vi "ecg_ncs_v3.vi"() -> ()   [LabVIEW 2016]
uses:
  <instrlib>/niUSRP/niUSRP Timestamp.ctl
  C:/Program Files/National Instruments/LabVIEW 2016/examples/Instrument IO/Serial/support/Serial - Settings.ctl
  State.ctl
  <vilib>/Instr/_visa.llb/VISA Configure Serial Port (Instr).vi
  <instrlib>/niUSRP/niUSRP Write Tx Data (2D CDB).vi
  <instrlib>/niUSRP/niUSRP Fetch Rx Data (2D CDB).vi
panel:
  in  "File Name 2":string="Test"
  in  "Path 2":path=path "D:/Research/SummerFall17Spring18/CnC/NCS/EcgNcsCorrelation/Labview Codes/ECG_NCS"
  out "#Loop = #Packets Received":i32
  out "ECGsample":i16
  out "PhNcs":dbl
  out "AmpNcs":dbl
  out "AmpNcsDS":dbl
  out "PhNcsDS":dbl
  out "error IO 2":errorcluster={"status"=FALSE, "code"=-1074118647, "source"=""}
  in  "Serial Settings":T1={"baud rate"=57600, "data bits"=8, "parity"=enum."None", "stop bits"=10, "flow control"=0} {"flow control" items=["None"=0, "XON/XOFF"=1, "RTS/CTS"=2, "DTR/DSR"=4]; "stop bits" items=["1.0"=10, "1.5"=15, "2.0"=20]; "data bits" min=5 max=8 step=1; "baud rate" items=["75"=75, "110"=110, "134"=134, "150"=150, "300"=300, "600"=600, "1200"=1200, "1800"=1800, "2400"=2400, "4800"=4800, "7200"=7200, "9600"=9600, "14400"=14400, "19200"=19200, "28800"=28800, "38400"=38400, "56000"=56000, "57600"=57600, "115200"=115200, "128000"=128000, "230400"=230400]}
  in  "VISA resource name":refnum<visa-resource-name>="bmd101"
  out "ECG":i16(graph)
  in  "byte count":u32=1
  out "Coerced Rx IQ Rate":dbl
  in  "Sampling Rate":i32=500
  out "Gain":dbl=-15.0
  out "Bandwidth":dbl=56000000.0
  out "Coerced Carrier Frequency":dbl=2000000000.0 format="%#.17g"
  out "Coerced Tx IQ rate":dbl=1000000.0
  out "error IO":errorcluster={"status"=FALSE, "code"=-1074118647, "source"=""}
  in  "Rx Number of Samples":i32=10000
  in  "Tab Control 2":enum32{"NI-294x/295x", "NI-2900/2901"}(tab)=enum."NI-2900/2901"
  in  "Rx carrier frequency [Hz]":dbl=2000000000.0 format="%#_6p"
  in  "Tx carrier frequency [Hz]":dbl=1000000000.0 format="%#_6p"
  in  "Start Trigger Time":T2={"whole seconds"=1, "fractional seconds"=0.0}
  in  "Tab Control":T3(tab)
  out "NCS tag Amp":dbl[](graph)=[0.011967714738528729, 0.012021355192189592, 0.012015275039596582, 0.011969166030167903, 0.011958890166168242, 0.012007893820858737, 0.012022893722444085, 0.011978222225113794, 0.011969989939463181, 0.012003099640895068]
  out "NCS tag Phase":dbl[](graph)=[0.011967714738528729, 0.012021355192189592, 0.012015275039596582, 0.011969166030167903, 0.011958890166168242, 0.012007893820858737, 0.012022893722444085, 0.011978222225113794, 0.011969989939463181, 0.012003099640895068]
  out "Tag Amp":dbl[](graph)
  out "Tag Phase":dbl[](graph)
  out "Tx Waveform Graph":waveform(dbl)[](graph)
  in  "Stop":bool
  in  "Channel 0\nTone Amplitude":dbl=0.707 step=0.05 format="%#.6g"
  in  "Channel 0 \nTone Frequency":dbl=5000.0 format="%#_6p"
  in  "Tx Waveform Size":dbl=2000.0
  in  "Device Name":refnum<k15>="MyB200"
  in  "Tx Gain":dbl=28.0 format="%#_6f"
  in  "Tx IQ Rate":dbl=1000000.0 format="%#_6p"
  in  "Rx Gain":dbl=32.0 format="%#_6f"
  in  "Rx IQ Rate":dbl=1000000.0 format="%#_6p"
  # "Rx Settings"
  # "Tx Settings"
  # "Note that on the NI-2900 and NI-2901, both Rx channels share an LO and both Tx channels share an LO. However, on the NI-294x/295x devices, Rx and Tx of channel 0 share an LO and Rx and Tx of channel 1 share an LO."
  # "Rx: Number of samples should be 1e6/512 in one loop."
  # "This Tx graph should always have end and start tied up since this is being sent in a loop continuously. Otherwise phase jumps will be noticed."
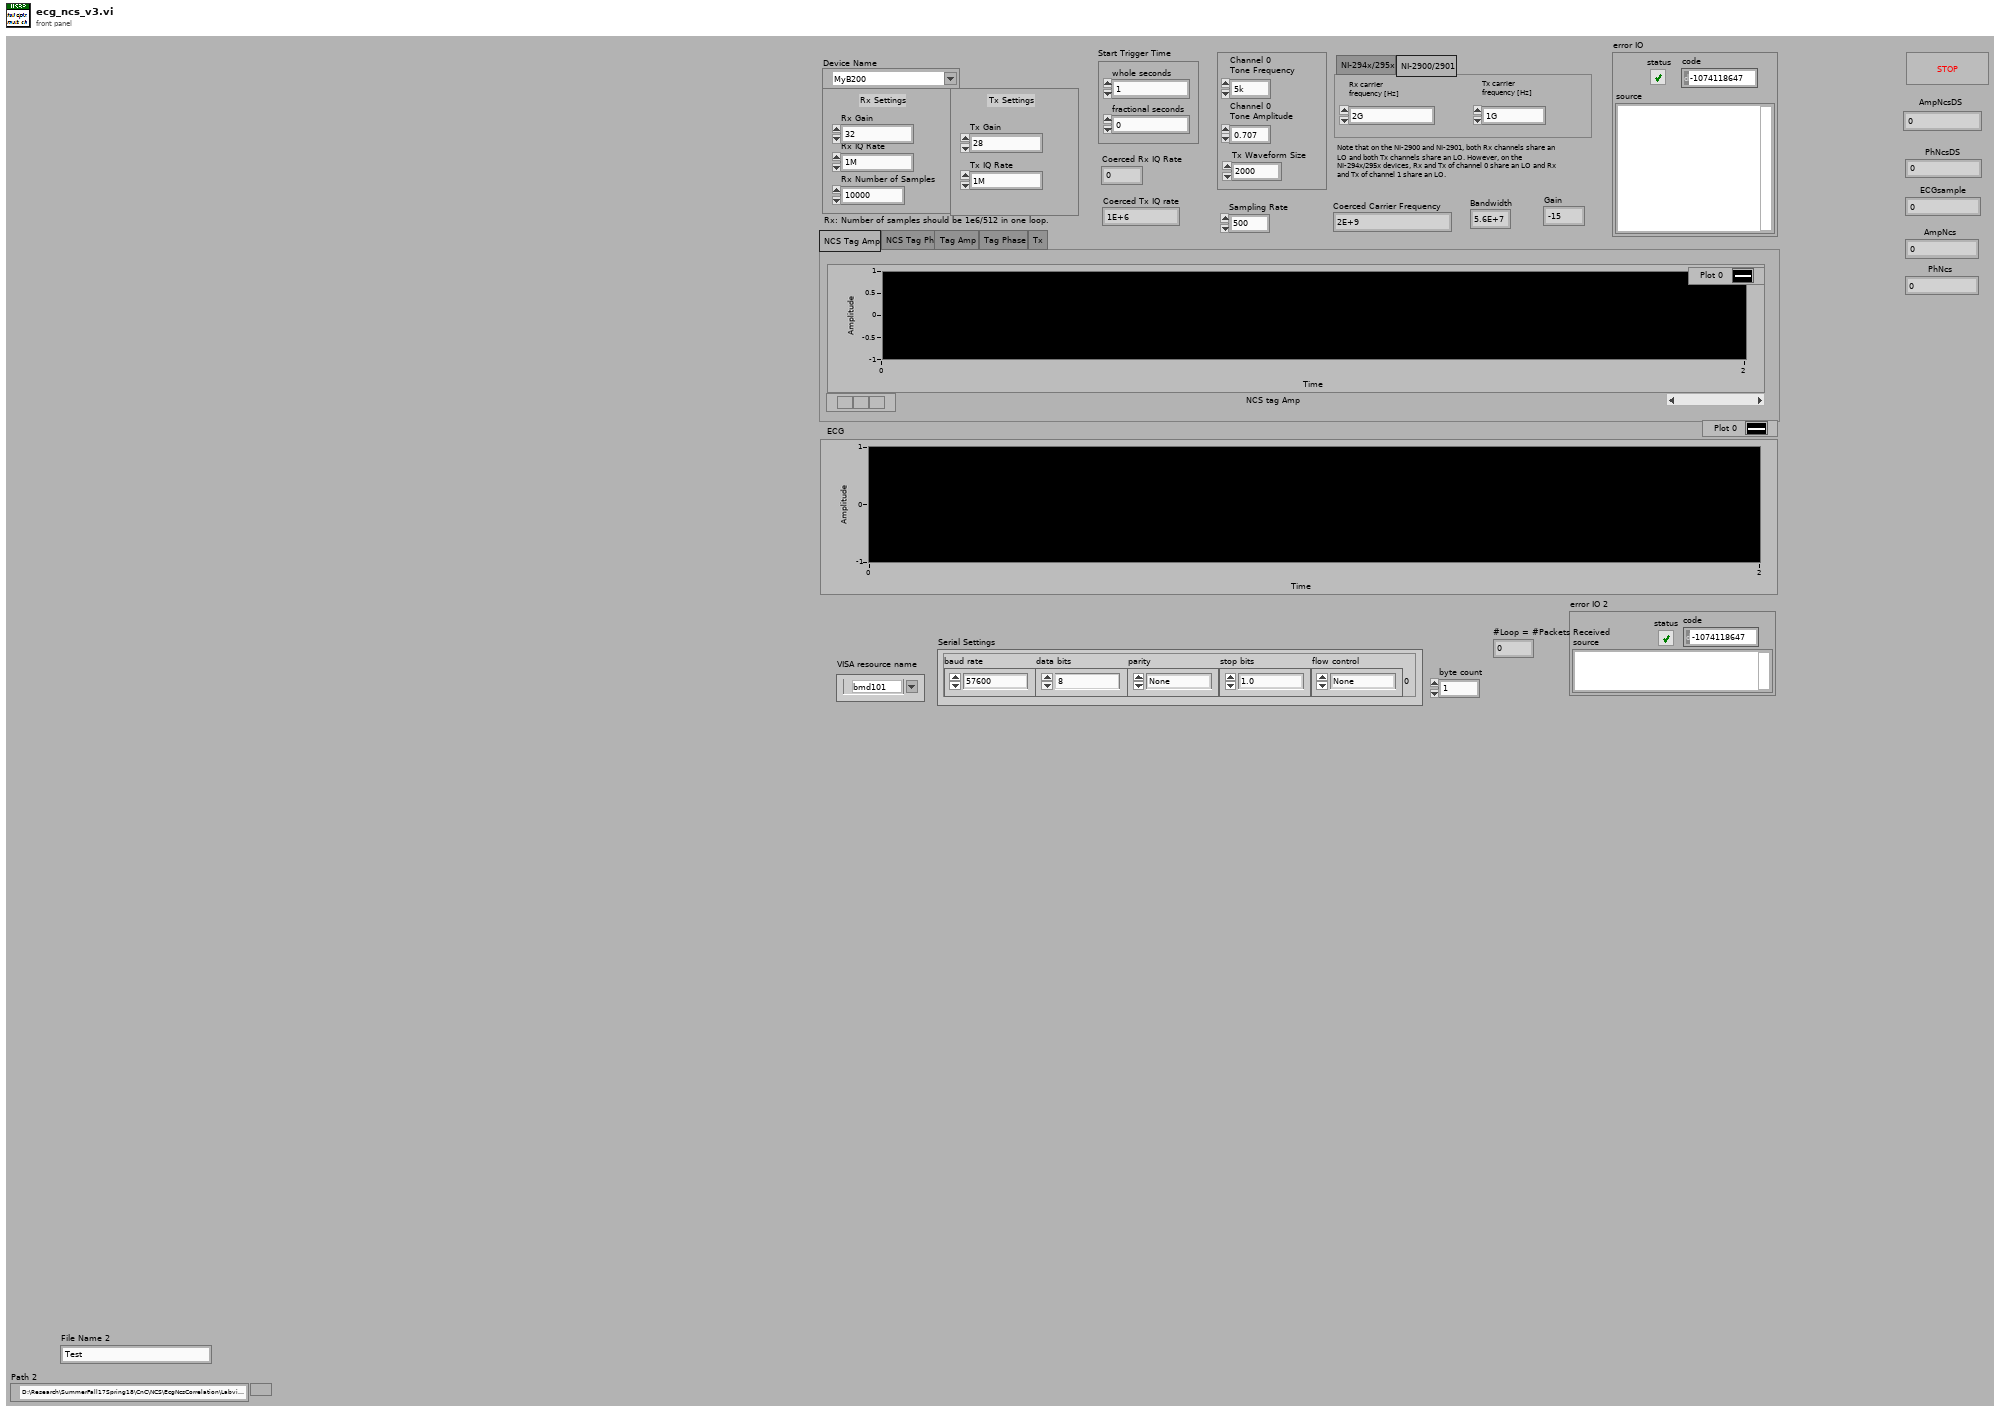
[diagram p1: front panel]
types:
  T1 = typedef "Serial - Settings.ctl" = cluster{"baud rate":u32, "data bits":u16, "parity":enum16{"None", "Odd", "Even", "Mark", "Space"}, "stop bits":u16, "flow control":u16}
  T2 = typedef "niUSRP Timestamp.ctl" = cluster{"whole seconds":u64, "fractional seconds":dbl}
  T3 = enum32{"NCS Tag Amp", "NCS Tag Ph", "Tag Amp", "Tag Phase", "Tx"}
  T4 = typedef "State.ctl" = enum16{"Initialize", "get byte", "check", "packet received", "packet approved"}
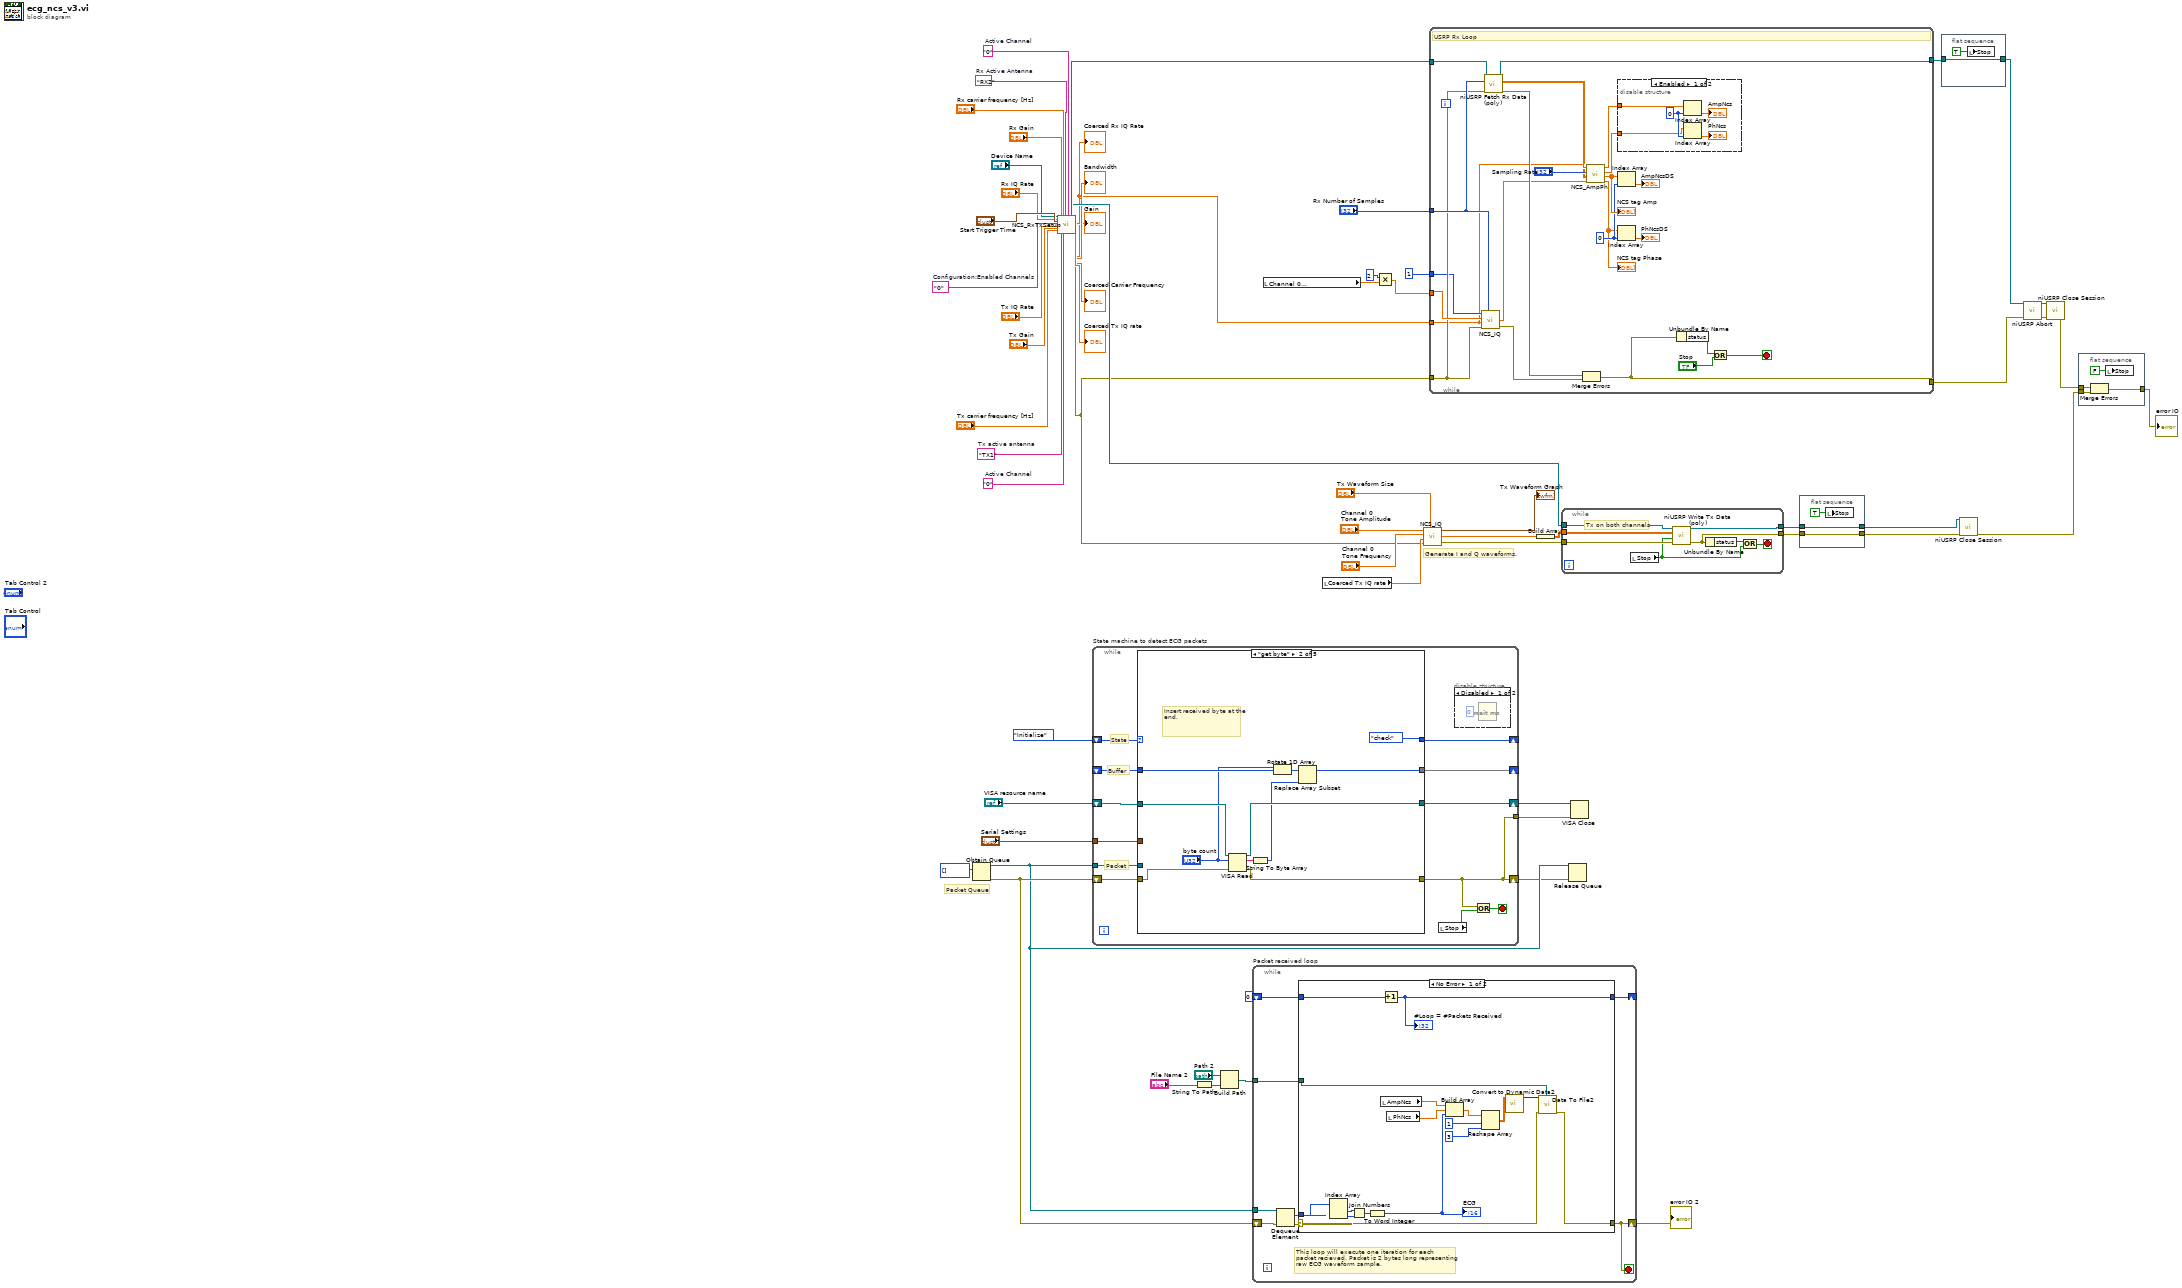
[diagram p0: block diagram]
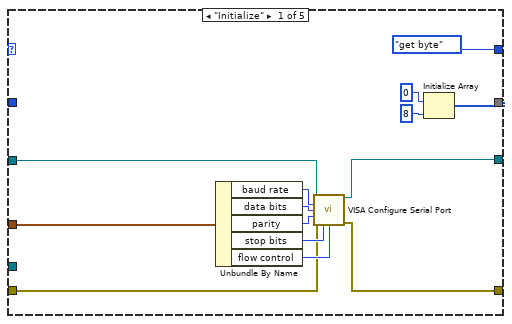
[diagram p4: hidden frame]
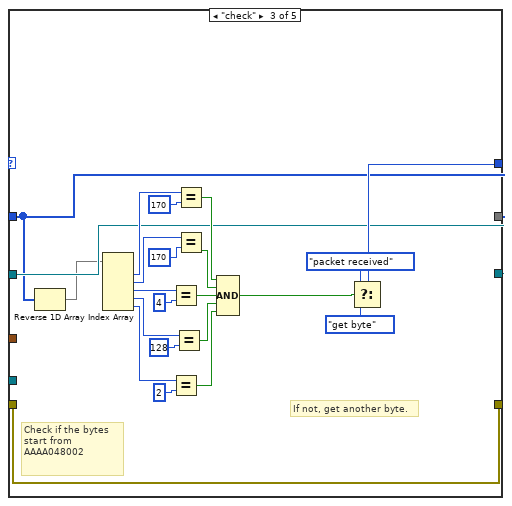
[diagram p5: hidden frame]
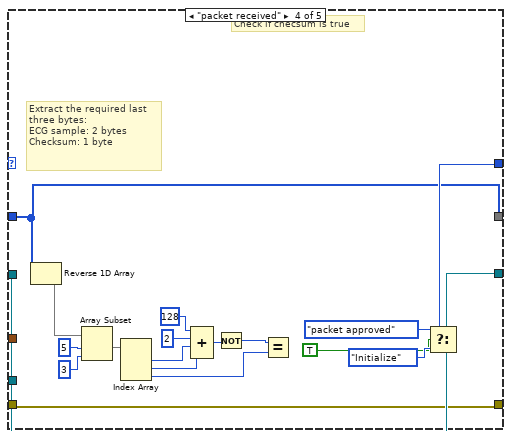
[diagram p6: hidden frame]
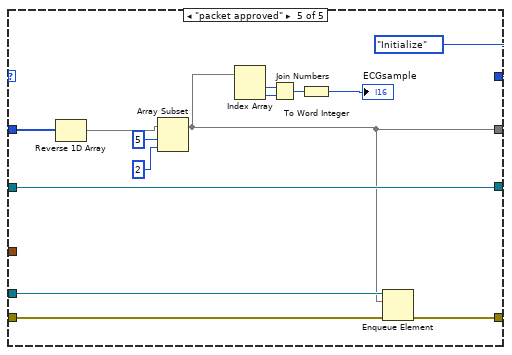
[diagram p7: hidden frame]
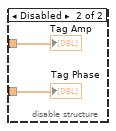
[diagram p8: hidden frame]
diagram:
  w17 = "0"  # Active Channel
  w18 = "0"  # Active Channel
  w53 = "RX2"  # Rx Active Antenna
  w49 = "TX1"  # Tx active antenna
  w35 = "0"  # Configuration:Enabled Channels
  # "Packet Queue"
  # "Generate I and Q waveforms."
  n1 = Obtain Queue(element data type=u8[] []) -> (queue out=w12:refnum<queue>, error out=w13:errorcluster)  [unwired: 4 in, 1 out]
  n2 = call "NCS_RxTxSetup.vi"("IVI Refnum in"="Device Name", "Rx IQ Rate"="Rx IQ Rate", "Start Trigger Time"="Start Trigger Time", "Configuration:Enabled Channels"=w35, "Tx IQ Rate"="Tx IQ Rate", "Tx Gain"="Tx Gain", "Tx carrier frequency [Hz]"="Tx carrier frequency [Hz]", "Rx Gain"="Rx Gain", "Tx active antenna"=w49, "Rx carrier frequency [Hz]"="Rx carrier frequency [Hz]", "Active Channel"=w17, "Rx Active Antenna"=w53, "Active Channel 2"=w18) -> ("session handle out"=w60:refnum<k15>, "IVI Refnum out"=w61:refnum<k15>, "Coerced Rx IQ Rate"=w16:dbl, "Bandwidth"=→"Bandwidth":dbl, "Gain"=→"Gain":dbl, "Carrier Frequency"=→"Coerced Carrier Frequency":dbl, "IQ Rate 2"=→"Coerced Tx IQ rate":dbl, "error out"=w28:errorcluster)  [unwired: 7 in]
  "Coerced Rx IQ Rate" <- w16
  n3 = while "State machine to detect ECG packets" {
    shift-right: [w64] -> w7
    shift-left: w13 -> [w70]
    shift-right: [w73] -> _
    shift-left: State."Initialize" ("State") -> [w72]
    shift-right: [w69] -> _
    shift-left: _ -> [w71]
    tunnel: w12 -> [w68]
    shift-right: [w67] -> w8
    shift-left: "VISA resource name" -> [w66]
    tunnel: "Serial Settings" -> [w65]
    tunnel: [w64] -> w6
    stop <- w63 stop-if-true
    # "State"
    # "Buffer"
    # "Packet"
    n4 = case shown="\"get byte\"" w72 {
      tunnel: [w85 w97 w101 w124 w143] -> w69
      tunnel: [State."get byte" ("State") State."check" ("f") w121 w130 State."Initialize" ("State")] -> w73
      tunnel: w71 -> [_ w90 w101 w124 w147]
      tunnel: w70 -> [w79 w94 w122 w131 w150]
      tunnel: [w78 w93 w122 w131 w149] -> w64
      tunnel: w68 -> [_ _ _ _ w151]
      tunnel: [w77 w95 w102 w138 w148] -> w67
      tunnel: w66 -> [w76 w96 w102 w138 w148]
      tunnel: w65 -> [w75 _ _ _ _]
      frame "Initialize" {
        n5 = Unbundle By Name(w75) -> ("baud rate"=w84:u32, "data bits"=w83:u16, "parity"=w82:enum16{"None", "Odd", "Even", "Mark", "Space"}, "stop bits"=w81:u16, "flow control"=w80:u16)
        n6 = call-poly "VISA Configure Serial Port"("VISA resource name"=w76, "baud rate (9600)"=w84, "data bits (8)"=w83, "parity (0:none)"=w82, "error in (no error)"=w79, "stop bits (10: 1 bit)"=w81, "flow control (0:none)"=w80) -> ("VISA resource name out"=w77:refnum<visa-resource-name>, "error out"=w78:errorcluster)  [unwired: 3 in, 4 out]
        n7 = Initialize Array(u8 0, 8 ("dimension size")) -> (w85:u8[])
      }
      frame "get byte" {
        # "Insert received byte at the end."
        n8 = VISA Read(VISA resource name=w96, byte count="byte count", error in (no error)=w94) -> (VISA resource name out=w95:refnum<visa-resource-name>, read buffer=w92:string, error out=w93:errorcluster)  [unwired: 1 out]
        n9 = String To Byte Array(string=w92) -> (unsigned byte array=w91:u8[])
        n10 = Rotate 1D Array(1:w90, 2:"byte count") -> (0:w98:u8[])
        n11 = Replace Array Subset(array=w98, new element=w91) -> (w97:u8[])  [unwired: 1 in]
      }
      frame "check" {
        # "If not, get another byte."
        # "Check if the bytes start from AAAA048002"
        n12 = Reverse 1D Array(array=w101) -> (reversed array=w100:u8[])
        n13 = Index Array(array=w100) -> (element #1=w108:u8, element #2=w107:u8, element #3=w106:u8, element #4=w105:u8, element #5=w104:u8)  [unwired: 5 in]
        n14 = Equal?(x=w106, y=u8 4 ("element")) -> (x = y?=w111:bool)
        n15 = Equal?(x=w104, y=u8 2 ("element")) -> (x = y?=w109:bool)
        n16 = Equal?(x=w105, y=u8 128 ("element")) -> (x = y?=w110:bool)
        n17 = Equal?(x=w108, y=u8 170 ("element")) -> (x = y?=w113:bool)
        n18 = Equal?(x=w107, y=u8 170 ("element")) -> (x = y?=w112:bool)
        n19 = Compound Arithmetic op=AND(w113, w112, w111, w110, w109) -> (w103:bool)
        n20 = Select(t=State."packet received" ("f"), s=w103, f=State."get byte") -> (s? t:f=w121:T4)
      }
      frame "packet received" {
        # "Check if checsum is true"
        # "Extract the required last three bytes: \nECG sample: 2 bytes\nChecksum: 1 byte"
        n21 = Reverse 1D Array(array=w124) -> (reversed array=w123:u8[])
        n22 = Array Subset(array=w123, index=5, length=3 ("index")) -> (w137:u8[])
        n23 = Index Array(array=w137) -> (element #1=w132:u8, element #2=w133:u8, element #3=w134:u8)  [unwired: 3 in]
        n24 = Compound Arithmetic op=ADD(u8 128 ("element"), u8 2 ("element"), w132, w133) -> (w127:u8)
        n25 = Not(x=w127) -> (.not. x?=w126:u8)
        n26 = Equal?(x=w126, y=w134) -> ()  [unwired: 1 out]
        n27 = Select(t=State."packet approved" ("State"), s=TRUE, f=State."Initialize" ("State")) -> (s? t:f=w130:T4)
      }
      frame "packet approved" {
        n28 = Reverse 1D Array(array=w147) -> (reversed array=w146:u8[])
        n29 = Array Subset(array=w146, index=5, length=2 ("index")) -> (w143:u8[])
        n30 = Index Array(array=w143) -> (element #1=w142:u8, element #2=w144:u8)  [unwired: 2 in]
        n31 = Join Numbers(hi=w142, lo=w144) -> ((hi.lo)=w145:u16)
        n32 = To Word Integer(number=w145) -> (16bit integer=→"ECGsample":i16)
        n33 = Enqueue Element(queue=w151, element=w143, error in (no error)=w150) -> (error out=w149:errorcluster)  [unwired: 1 in, 2 out]
      }
    }
    n34 = local read "Stop"() -> (w62:bool)
    n35 = disable-structure shown="Disabled" {
      frame Disabled {
        n36 = Wait (ms)(milliseconds to wait=u32 0) -> ()  [unwired: 1 out]
      }
      frame Enabled {
      }
    }
    n37 = Or(x=w64, y=w62) -> (x .or. y?=w63:bool)
  }
  n38 = String To Path(string="File Name 2") -> (path=w4:path)
  n39 = Build Path(base path="Path 2", name or relative path=w4) -> (appended path=w1:path)
  n40 = while "Packet received loop" {
    shift-right: [w158] -> w9
    shift-left: w13 -> [w162]
    tunnel: w12 -> [w161]
    shift-right: [w156] -> _
    shift-left: 0 -> [w157]
    tunnel: w1 -> [w155]
    stop <- w158 stop-if-true
    # "This loop will execute one iteration for each\npacket recieved. Packet is 2 bytes long representing \nraw ECG waveform sample."
    n41 = Dequeue Element(queue=w161, error in (no error)=w162) -> (element=w160:u8[], error out=w159:errorcluster)  [unwired: 1 in, 2 out]
    n42 = case shown="No Error" w159 {
      selector: w159 -> [w166 w181]
      tunnel: w160 -> [w179 _]
      tunnel: [w165 w181] -> w158
      tunnel: w157 -> [w175 w180]
      tunnel: [w174 w180] -> w156
      tunnel: w155 -> [w168 _]
      frame No Error {
        n43 = Index Array(array=w179) -> (element #1=w178:u8, element #2=w177:u8)  [unwired: 2 in]
        n44 = Join Numbers(hi=w178, lo=w177) -> ((hi.lo)=w176:u16)
        n45 = To Word Integer(number=w176) -> (16bit integer=w167:i16)
        "ECG" <- w167
        n46 = local read "AmpNcs"() -> (w164:dbl)
        n47 = Increment(x=w175) -> (x+1=w174:i32)
        "#Loop = #Packets Received" <- w174
        n48 = local read "PhNcs"() -> (w163:dbl)
        n49 = Build Array(w164, w163, w167) -> (w172:dbl[])
        n50 = Reshape Array(w172, 1 ("dimension size"), 3 ("dimension size")) -> (w169:dbl[][])
        n51 = call "Convert to Dynamic Data2"("2D Array"=w169) -> ("Dynamic Data Type"=w173:dynamicdata)  [unwired: 3 in]
        n52 = call "Data To File2"("Signals"=w173, "error in (no error)"=w166, "Filename"=w168) -> ("error out"=w165:errorcluster)  [unwired: 14 in, 2 out]
      }
      frame Error {
      }
    }
  }
  "error IO 2" <- w9
  n53 = local read "Channel 0 \nTone Frequency"() -> (w34:dbl)
  n54 = local read "Coerced Tx IQ rate"() -> (w29:dbl)
  n55 = Multiply(x=2, y=w34) -> (x*y=w33:dbl)
  n56 = call "NCS_IQ.vi"("Tone Amplitude"="Channel 0\nTone Amplitude", "Waveform Size"="Tx Waveform Size", "Tone Frequency"="Channel 0 \nTone Frequency", "Coerced IQ rate"=w29, "error in (no error)"=w28) -> ("IQ waveform"=→"Tx Waveform Graph":waveform(dbl)[], "IQ waveform array"=w26:cdb[], "error out"=w27:errorcluster)  [unwired: 1 in]
  n57 = while {
    tunnel: w61 -> [w204]
    tunnel: w28 -> [w197]
    tunnel: [w203] -> w45
    tunnel: "Rx Number of Samples" -> [w199]
    tunnel: w16 -> [w193]
    tunnel: [w194] -> w37
    tunnel: w33 -> [w198]
    tunnel: 1 -> [w195]
    stop <- w200 stop-if-true
    w185 = 0
    # "USRP Rx Loop"
    n58 = call "NCS_IQ.vi"("Tone Amplitude"=w195, "Waveform Size"=w199, "Tone Frequency"=w198, "Coerced IQ rate"=w193, "error in (no error)"=w197) -> ("IQ waveform array"=w190:cdb[], "error out"=w196:errorcluster)  [unwired: 1 in, 1 out]
    n59 = call-poly <instrlib>:"niUSRP Fetch Rx Data (poly).vi"("session handle"=w204, "number of samples"=w199, "error in (no error)"=w197) -> ("session handle out"=w203:refnum<k15>, "data"=w191:cdb[][], "error out"=w201:errorcluster)  [unwired: 9 in, 1 out]
    n60 = Merge Errors(w201, w196) -> (w194:errorcluster)
    n61 = call "NCS_AmpPh.vi"("IQ"=w190, "data"=w191, "Sampling Rate"="Sampling Rate", "Coerced Rx IQ Rate"=w193) -> ("Phase DownSampled"=w184:dbl[], "Amp DownSampled"=w186:dbl[], "Phase"=w188:dbl[], "Amplitude"=w189:dbl[])  [unwired: 4 in]
    "NCS tag Amp" <- w186
    "NCS tag Phase" <- w184
    n62 = disable-structure shown="Enabled" {
      disable-tunnel: w189 -> [w208 w211]
      disable-tunnel: w188 -> [w207 w210]
      frame Enabled {
        w209 = 0
        n63 = Index Array(array=w208, index=w209) -> (element=→"AmpNcs":dbl)
        n64 = Index Array(array=w207, index=w209) -> (element=→"PhNcs":dbl)
      }
      frame Disabled {
        "Tag Amp" <- w211
        "Tag Phase" <- w210
      }
    }
    n65 = Index Array(array=w186, index=w185) -> (element=→"AmpNcsDS":dbl)
    n66 = Index Array(array=w184, index=w185) -> (element=→"PhNcsDS":dbl)
    n67 = Unbundle By Name(w194) -> ("status"=w202:bool)
    n68 = Or(x=w202, y="Stop") -> (x .or. y?=w200:bool)
  }
  n69 = Build Array(w26) -> (w57:cdb[][])
  n70 = while {
    tunnel: w60 -> [w219]
    tunnel: w27 -> [w218]
    tunnel: [w216] -> w48
    tunnel: [w214] -> w43
    tunnel: w57 -> [w212]
    stop <- w215 stop-if-true
    # "Tx on both channels"
    n71 = local read "Stop"() -> (w213:bool)
    n72 = call-poly <instrlib>:"niUSRP Write Tx Data (poly).vi"("session handle"=w219, "data"=w212, "end of data?"=w213, "error in (no error)"=w218) -> ("session handle out"=w214:refnum<k15>, "error out"=w216:errorcluster)  [unwired: 10 in]
    n73 = Unbundle By Name(w216) -> ("status"=w217:bool)
    n74 = Compound Arithmetic op=OR(w217, w213) -> (w215:bool)
  }
  n75 = Release Queue(queue=w12, error in (no error)=w7) -> ()  [unwired: 1 in, 3 out]
  n76 = VISA Close(VISA resource name=w8, error in (no error)=w6) -> ()  [unwired: 1 out]
  n77 = flat-sequence {
    tunnel: [w221] -> w47
    tunnel: w48 -> [w221]
    tunnel: [w220] -> w44
    tunnel: w43 -> [w220]
    frame #0 {
      n78 = local write "Stop"(TRUE ("STOP")) -> ()
    }
  }
  n79 = flat-sequence {
    tunnel: [w223] -> w46
    tunnel: w45 -> [w223]
    frame #0 {
      n80 = local write "Stop"(TRUE ("STOP")) -> ()
    }
  }
  n81 = call <instrlib>:"niUSRP Close Session.vi"("session handle"=w44, "error in (no error)"=w47) -> ("error out"=w42:errorcluster)  [unwired: 13 in]
  n82 = call <instrlib>:"niUSRP Abort.vi"("session handle"=w46, "error in (no error)"=w37) -> ("session handle out"=w59:refnum<k15>, "error out"=w58:errorcluster)  [unwired: 12 in]
  n83 = call <instrlib>:"niUSRP Close Session.vi"("session handle"=w59, "error in (no error)"=w58) -> ("error out"=w39:errorcluster)  [unwired: 13 in]
  n84 = flat-sequence {
    tunnel: w42 -> [w227]
    tunnel: [w226] -> w40
    tunnel: w39 -> [w225]
    frame #0 {
      n85 = Merge Errors(w225, w227) -> (w226:errorcluster)
      n86 = local write "Stop"(FALSE ("STOP")) -> ()
    }
  }
  "error IO" <- w40
